vi "Shutdown.vi"(8 "error in (no error)":errorcluster, 11 "DbgTimers in":refnum<class "DbgTimers.lvclass">) -> (0 "error out":errorcluster, 3 "DbgTimers out":refnum<class "DbgTimers.lvclass">)   [LabVIEW 2017, in "DbgTimers.lvclass"]
doc: "Developed by Kevin Thompson\nkevin@thompsonengineering.net\n\nCopyright 2018-2020\nThompson Engineering, LLC"
uses:
  DbgTimers.lvclass
  DbgTimers.lvclass/DbgTimers.ctl
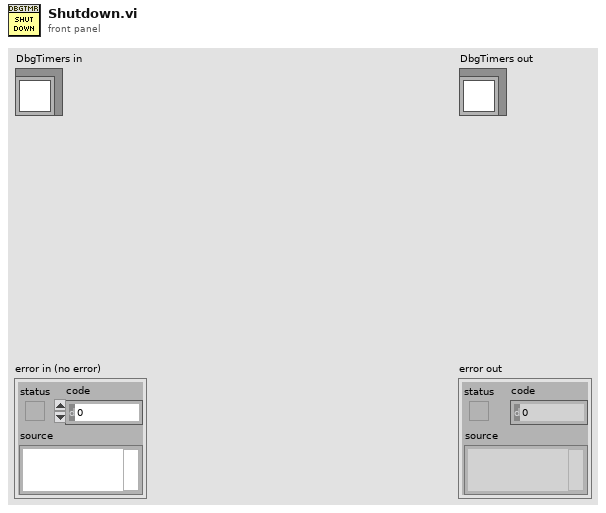
[diagram p1: front panel]
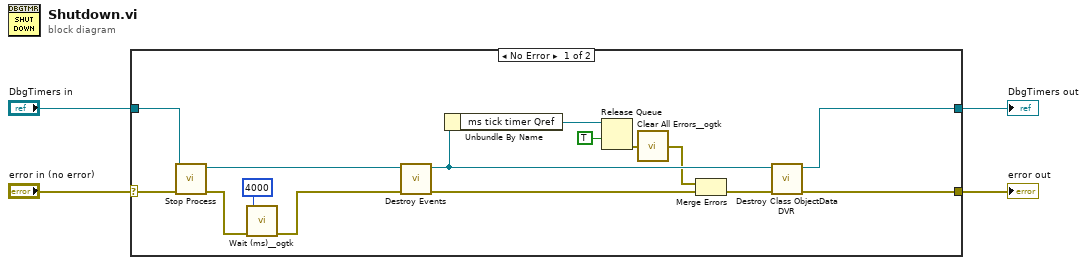
[diagram p0: block diagram]
diagram:
  n1 = case shown="No Error" "error in (no error)" {
    selector: "error in (no error)" -> [w19 w21]
    tunnel: [w16 w21] -> w3
    tunnel: [w15 w20] -> w1
    tunnel: "DbgTimers in" -> [w18 w20]
    frame No Error {
      n2 = call "Stop Process.vi"("error in (no error)"=w19, "DbgTimers in"=w18) -> ("error out"=w7:errorcluster, "DbgTimers out"=w17:refnum<class "DbgTimers.lvclass">)  [unwired: 8 in]
      n3 = call <userlib>:"Wait (ms)__ogtk.vi"("error in (no error)"=w7, "milliseconds to wait"=u32 4000) -> ("error out"=w6:errorcluster)  [unwired: 8 in, 1 out]
      n4 = call "Destroy Events.vi"("error in (no error)"=w6, "DbgTimers in"=w17) -> ("error out"=w11:errorcluster, "DbgTimers out"=w14:refnum<class "DbgTimers.lvclass">)  [unwired: 8 in]
      n5 = Unbundle By Name(w14) -> ("ms tick timer Qref"=w13:refnum<queue>)
      n6 = Release Queue(queue=w13, force destroy? (F)=TRUE) -> (error out=w9:errorcluster)  [unwired: 1 in, 2 out]
      n7 = call <userlib>:"Clear All Errors__ogtk.vi"("Error In"=w9) -> ("Error Out"=w8:errorcluster)  [unwired: 3 in]
      n8 = Merge Errors(w8, w11) -> (w10:errorcluster)
      n9 = call "Destroy Class ObjectData DVR.vi"("error in (no error)"=w10, "DbgTimers in"=w14) -> ("error out"=w16:errorcluster, "DbgTimers out"=w15:refnum<class "DbgTimers.lvclass">)  [unwired: 8 in]
    }
    frame Error {
    }
  }
  "error out" <- w3
  "DbgTimers out" <- w1
